vi "Main FPGA.vi"() -> ()   [LabVIEW 2015]
uses:
  Controls/FPGA_ACQTime State.ctl
  Controls/Phase State.ctl
  Controls/FPGA_Line Syn. State.ctl
  Controls/FPGA_Y AO State.ctl
  Controls/FPGA_Stimulate State.ctl
  <vilib>/Platform/TimedLoop/XDataNode/timing_clust.ctl
  <vilib>/Platform/TimedLoop/XDataNode/nitl_modes.ctl
  <vilib>/Platform/TimedLoop/XDataNode/wakeup.ctl
  Controls/FPGA_Enable Frame State.ctl
  <vilib>/rvi/Emulation/niFpgaGetClockAttributes.vi
  <vilib>/rvi/Emulation/niFpgaSctlEmulationGetInTimedLoop.vi
  <vilib>/rvi/Emulation/niFpgaEmulationReportErrorSimple.vi
  <vilib>/rvi/Emulation/niFpgaProcessEmulError.vi
  <vilib>/rvi/eio/common/nirviEmuTemplateMethod_errors.vi
  <vilib>/rvi/Emulation/niFpgaCriticalErrorInLSC.vi
  <vilib>/rvi/Memory/Memory_Emulation/nirvimemoryFastEmulation.vi
  <vilib>/rvi/Memory/Memory_Emulation/nirvimemoryEmulation.vi
  <vilib>/rvi/Emulation/niFpgaEmulationIsFPGAContextNoSignature.vi
  <vilib>/rvi/DataTransferAndStorage/Container/Common/niFpgaContainerGetUniqueNameForEmu.vi
  <vilib>/rvi/errors/nirviReportUnexpectedCaseInternalError (U32).vi
  <vilib>/rvi/interface/RandomDataEmulation/niFpgaRandomDataHandleErrors.vi
  <vilib>/eio/EIONode/EIONode.xnode
  <vilib>/rvi/DataTransferAndStorage/Container/XNode/niFpgaContainer.xnode
  <vilib>/Platform/TimedLoop/XDataNode/XDataNode.xnode
  <vilib>/rvi/interface/RandomDataEmulation/nirviRandomDataFpgaReadWriteTemplate.vi
  <instrlib>/_niInstr/Basic Elements/v1/FPGA/niInstr Basic Elements v1 FPGA.lvlib
  <vilib>/Platform/TimedLoop/XDataNode/XDNodeRunTimeDep.lvlib
panel:
  in  "PMT1 Enable":bool
  in  "Vision Stimulate Value":i16
  in  "Stimulate Enable":bool
  in  "Stimulate Time":u32
  in  "Stimulate Interval":u32
  in  "Frames Befor Stimulate":u32
  out "Frame Number":u32
  out "VSYNC":bool
  out "Actual Stimulate Ticks":u32
  out "Actual Laser Intensity":i16
  in  "Actual Laser Intensity Count":u32
  out "Acutal Actual Laser Intensity Count":u32
  in  "Y Offset":i16
  in  "Point":bool
  in  "Microscope":enum16{"Miniature", "Benchtop"}(ring)
  in  "Laser Intensity Count(Ticks)":u32 caption="PMT Sensitivity Count(Ticks)"
  out "Actual Laser Intensity Count(Ticks)":u32
  out "Acq. Syn. Out":bool
  in  "X Offset":i16
  in  "Laser Intensity":i16
  in  "Threh.Low":i16
  in  "Threh.High":i16
  in  "High Dealy":u32
  in  "Low Dealy":u32
  out "Actual PMT Sensitivity Count(Ticks)":u32
  in  "PMT Sensitivity Count(Ticks)":u32
  in  "PMT Sensitivity":i16
  in  "Start Control":bool
  out "2":i16
  out "1":i16
  out "Triangle 剩余元素":u32
  out "Ramp 剩余元素":u32
  out "IDLE":bool
  out "Ramp 待读取元素数量":u32
  out "Triangle 待读取元素数量":u32
  in  "Shutter":bool
  out "Falling Detected":bool
  out "Rising Detected":bool
  in  "Phase Shift":u32
  out "Acq. Time Number":u32
  out "Line Dis.":u32
  in  "Line":u32
  in  "Ramp Step":i16
  in  "Ramp Start":i16
  in  "Triangle Min":i16
  in  "Triangle Max":i16
  out "Ramp Number":u32
  out "Ramp OutEnable":bool
  out "Laser data out":i16
  in  "FPGA Stop":bool=TRUE
  out "Actual Wave Ticks":u32
  out "Triangle OutEnable":bool
  in  "Wave Ticks":u32
  out "Triangle Number":u32
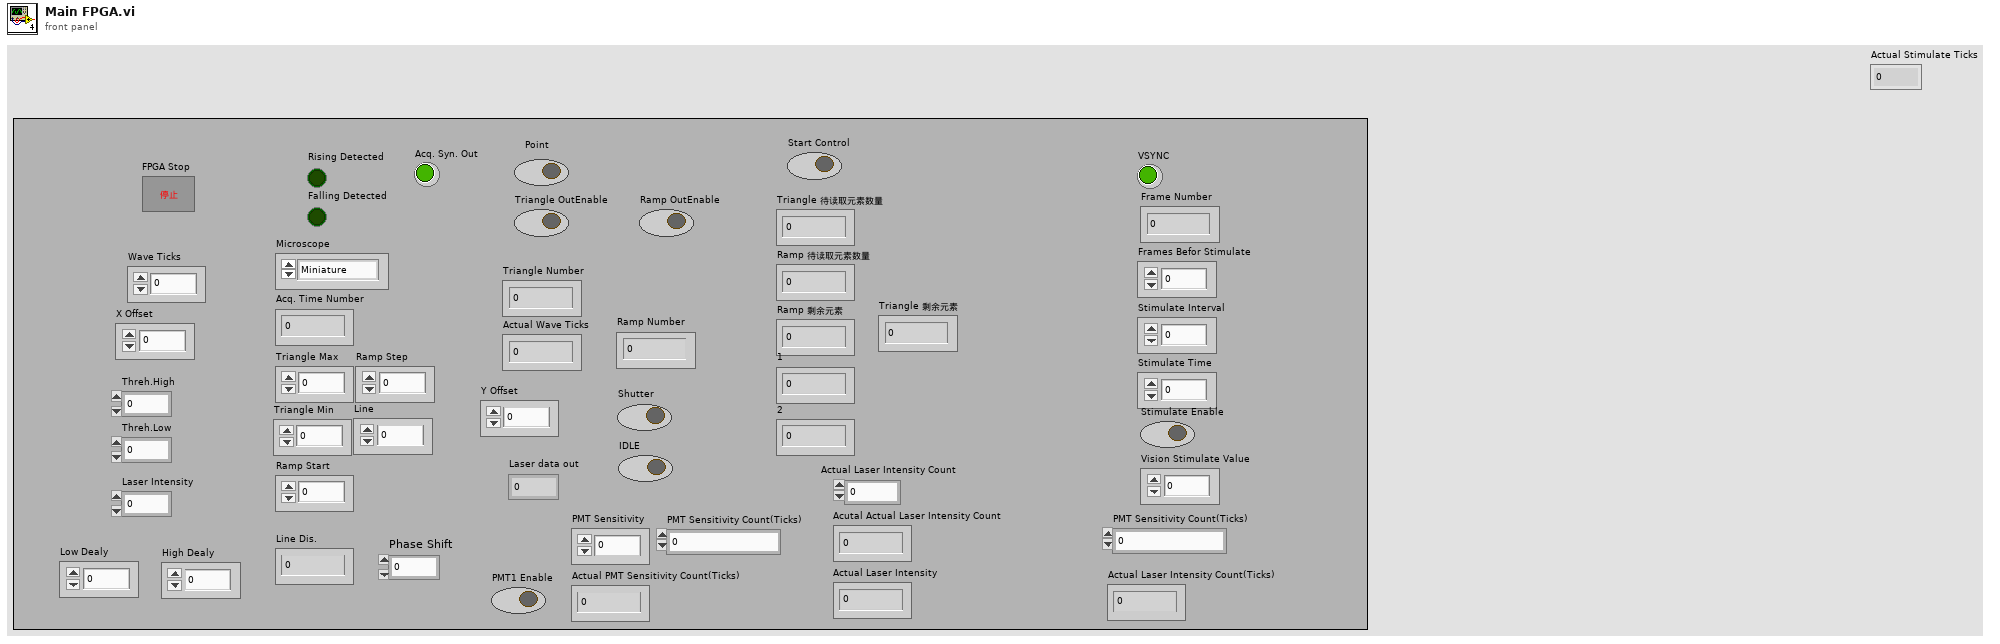
[diagram p1: front panel]
types:
  T1 = typedef "FPGA_Stimulate State.ctl" = enum16{"Wait Frame", "Frame Count", "Stiumalting", "Stiumlate Delay"}
  T2 = typedef "FPGA_Y AO State.ctl" = enum16{"Frame Start", "Framing", "Ramp"}
  T3 = typedef "FPGA_Line Syn. State.ctl" = enum16{"Wait Low", "Low Delay", "Wait High", "High Delay"}
  T4 = typedef "Phase State.ctl" = enum16{"Wait for Rising", "Wait for Falling ", "Rising Delay", "Falling Delay"}
  T5 = typedef "FPGA_ACQTime State.ctl" = enum16{"Init", "Rising Eadge", "Falling Eadge"}
  T6 = typedef "FPGA_Enable Frame State.ctl" = enum16{"Wait Enable", "Enable", "Output"}
  T7 = typedef "XDNodeRunTimeDep.lvlib/timing_clust.ctl" = cluster{"Expected End [f-1]":u64, "Actual End [f-1]":u64, "Finished Late? [f-1]":bool, "Expected End [i-1]":u64, "Actual End [i-1]":u64, "Finished Late? [i-1]":bool, "Expected Start [i]":u64, "Actual Start [i]":u64, "Expected Start [f]":u64, "Actual Start [f]":u64, "Source Name":string, "Structure Name":string, "Period":i64, "Deadline":i64, "Offset":i64, "Start":i64, "Priority":i32, "Timeout":i32, "Mode":T8, "Wakeup Reason":T9, "Error":errorcluster, "Source Type":string, "Secondary Source Type":string, "Global End Time":u64, "Global Start Time":u64, "Frame Duration":u64, "Iteration Duration":u64, "Assigned CPU":i32, "I/O Scan Engine Mode":u32}
  T8 = typedef "XDNodeRunTimeDep.lvlib/nitl_modes.ctl" = enum32{"No Change", "Process missed periods, maintain original phase", "Discard missed periods, maintain original phase", "Process missed periods, ignore original phase", "Discard missed periods, ignore original phase"}
  T9 = typedef "XDNodeRunTimeDep.lvlib/wakeup.ctl" = enum32{"Normal", "Aborted", "Asynchronous wakeup", "Timing source error", "Timed loop error", "Timeout"}
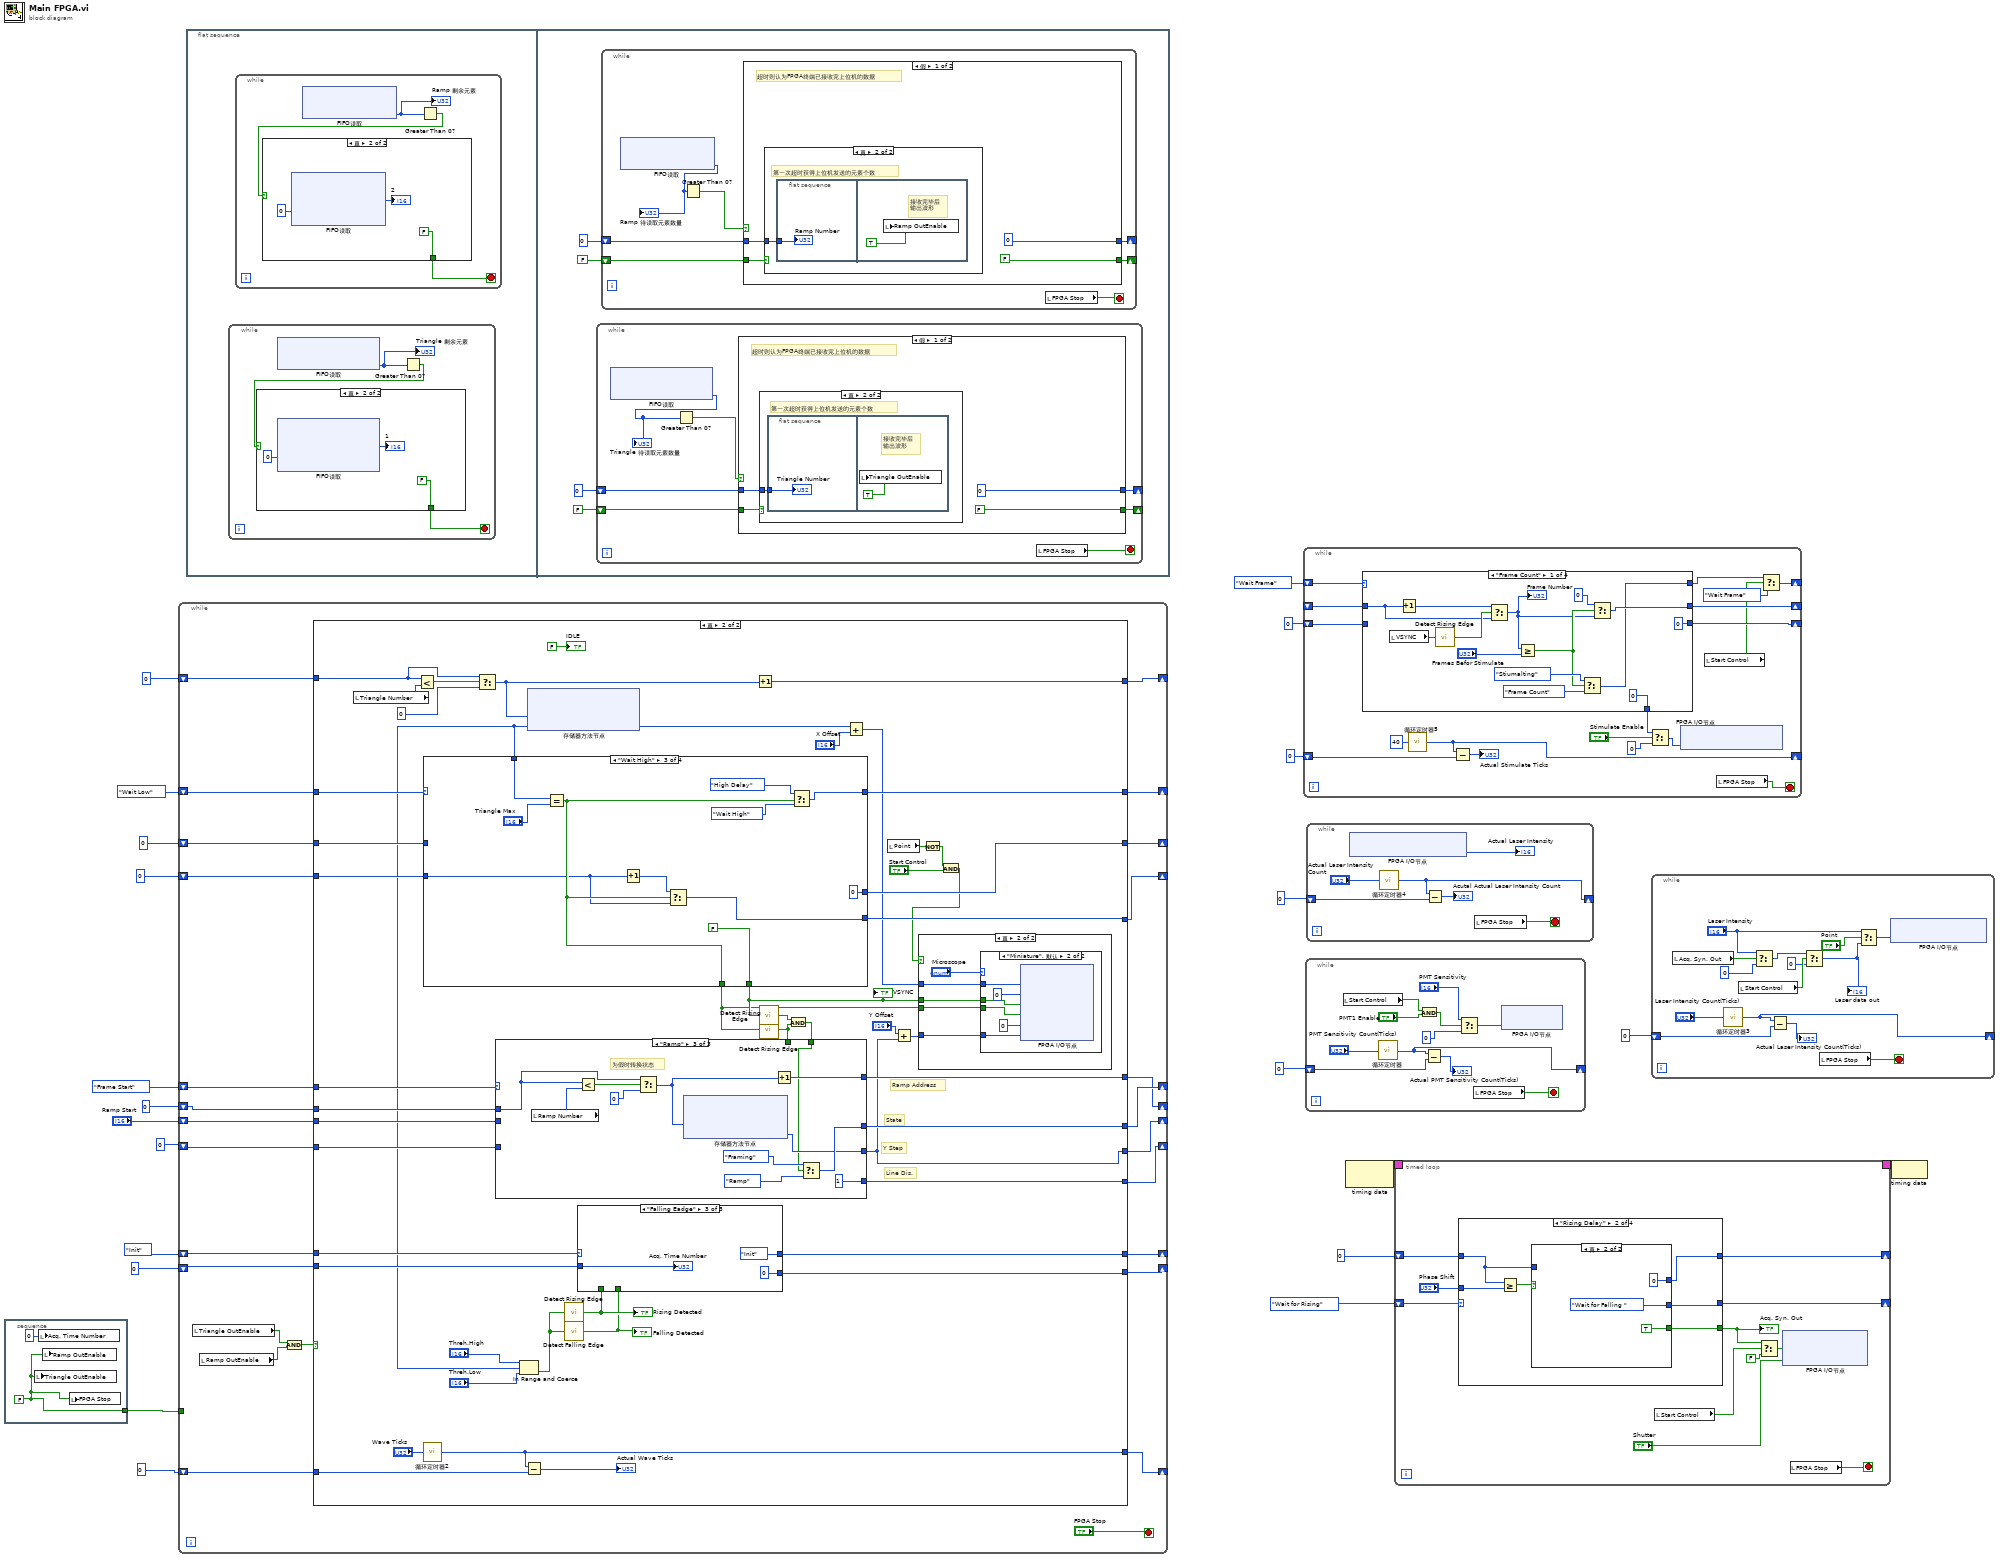
[diagram p0: block diagram]
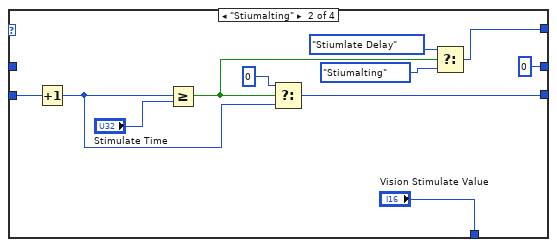
[diagram p2: hidden frame]
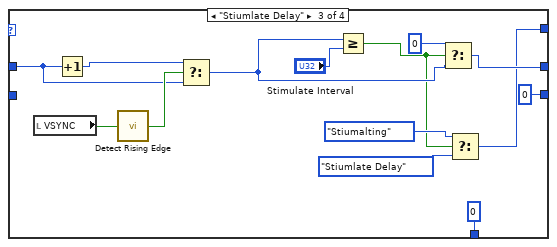
[diagram p3: hidden frame]
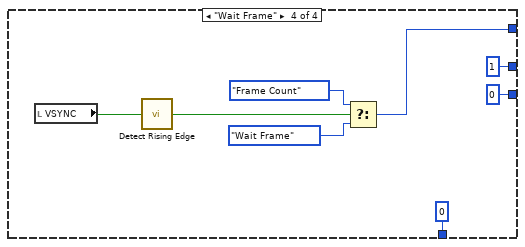
[diagram p4: hidden frame]
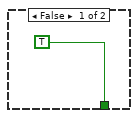
[diagram p5: hidden frame]
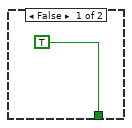
[diagram p6: hidden frame]
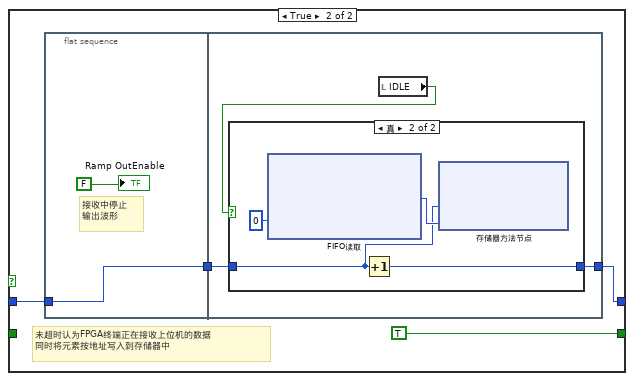
[diagram p8: hidden frame]
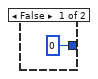
[diagram p9: hidden frame]
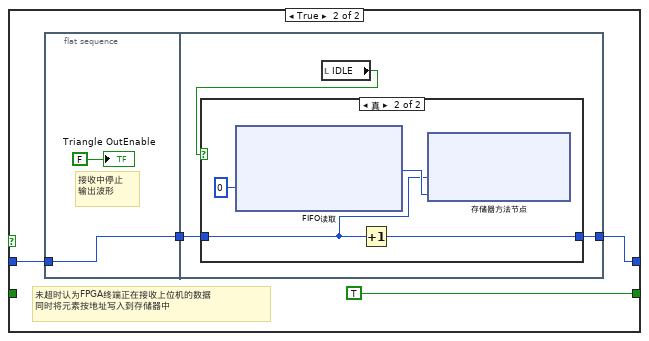
[diagram p11: hidden frame]
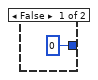
[diagram p12: hidden frame]
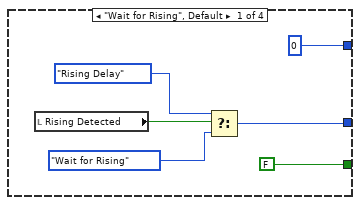
[diagram p13: hidden frame]
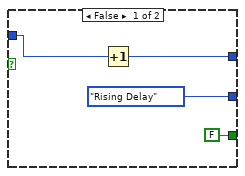
[diagram p14: hidden frame]
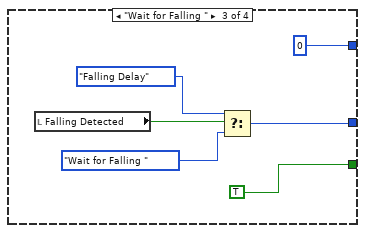
[diagram p15: hidden frame]
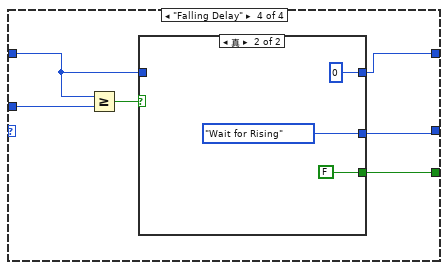
[diagram p16: hidden frame]
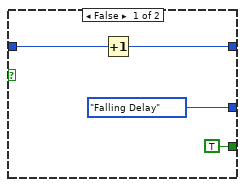
[diagram p17: hidden frame]
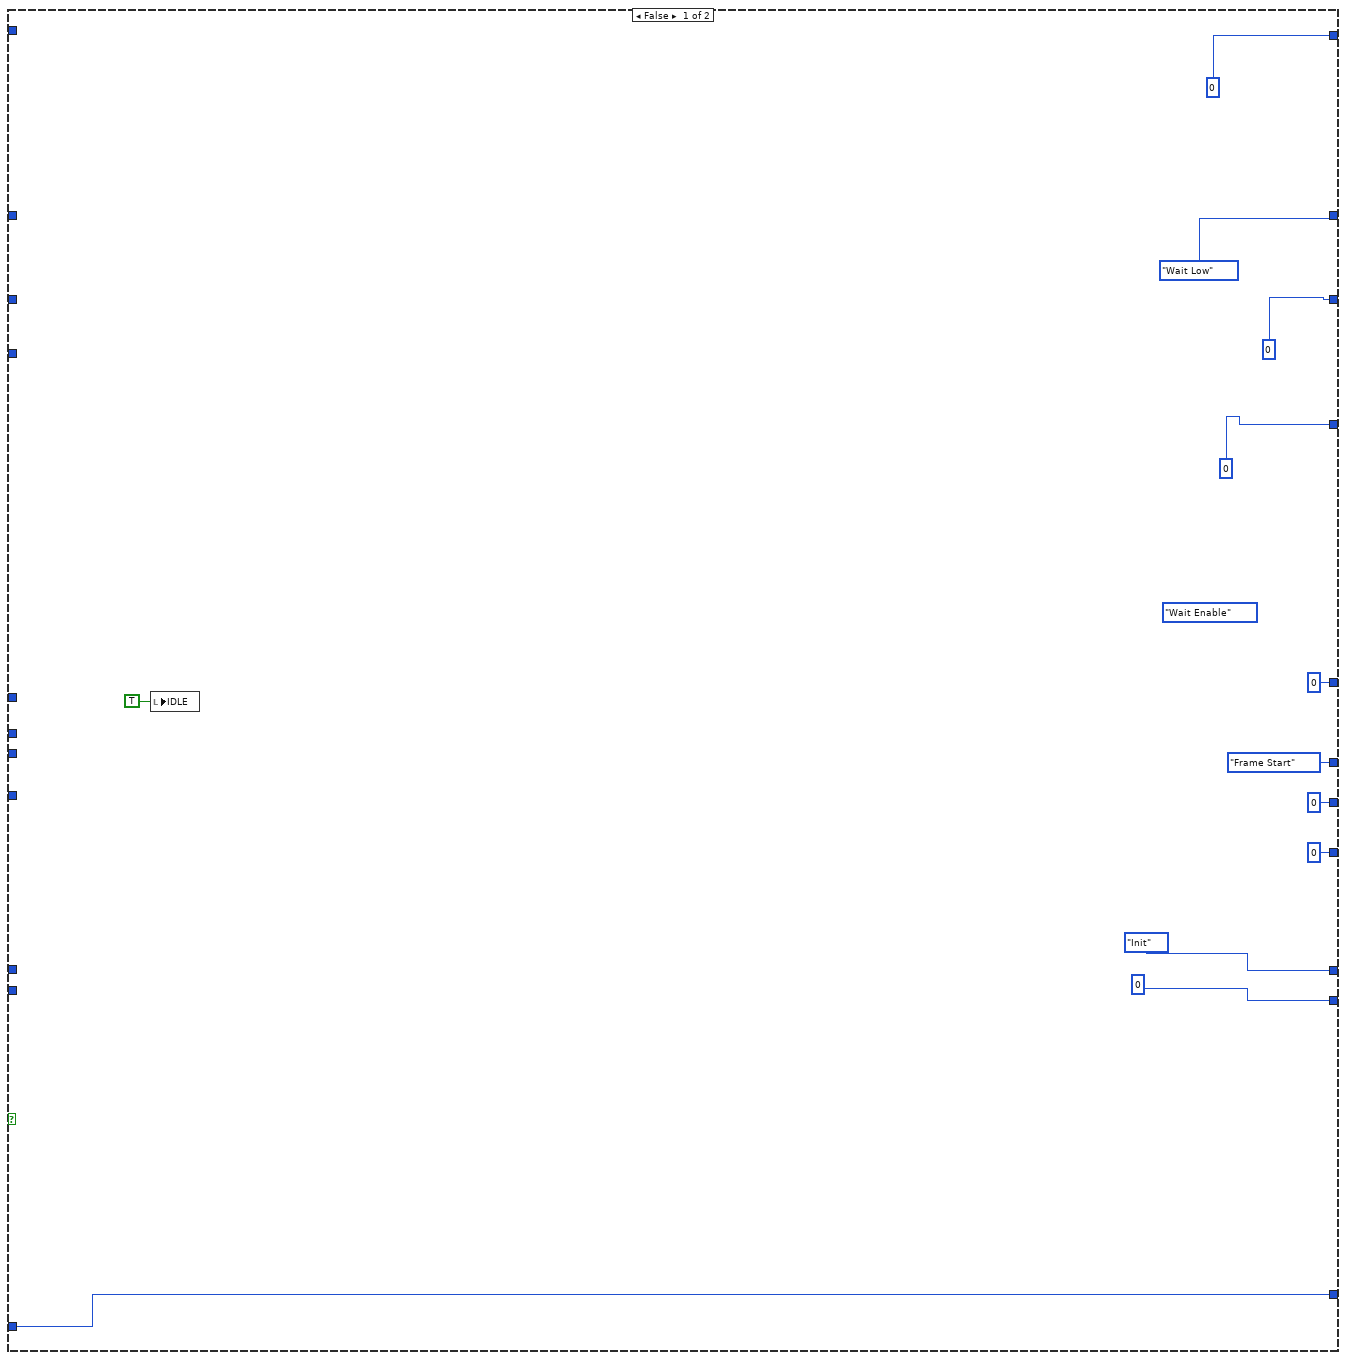
[diagram p18: hidden frame]
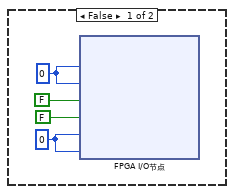
[diagram p19: hidden frame]
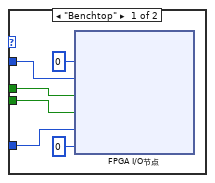
[diagram p20: hidden frame]
diagram:
  n1 = stacked-sequence {
    tunnel: [w24] -> w20
    frame #0 {
      w24 = FALSE ("FPGA Stop")
      n2 = local write "Triangle OutEnable"(w24) -> ()
      n3 = local write "Acq. Time Number"(u32 0 ("Acq. Time Number")) -> ()
      n4 = local write "Ramp OutEnable"(w24) -> ()
      n5 = local write "FPGA Stop"(w24) -> ()
    }
  }
  n6 = while {
    shift-right: [w50] -> _
    shift-left: u32 0 ("地址") -> [w49]
    shift-right: [w48] -> _
    shift-left: u32 0 ("地址") -> [w47]
    shift-right: [w37] -> _
    shift-left: FPGA_Line_Syn._State."Wait Low" ("Line Syn. State") -> [w45]
    tunnel: w20 -> [_]
    shift-right: [w40] -> _
    shift-left: FPGA_ACQTime_State."Init" ("FPGA_ACQTime State") -> [w41]
    shift-right: [w38] -> _
    shift-left: u32 0 ("地址") -> [w39]
    shift-right: [w35] -> _
    shift-left: u32 0 ("地址") -> [w36]
    shift-right: [w33] -> _
    shift-left: u32 0 ("地址") -> [w34]
    shift-right: [w31] -> _
    shift-left: FPGA_Y_AO_State."Frame Start" ("Y/AO State") -> [w32]
    shift-right: [w28] -> _
    shift-left: "Ramp Start" -> [w30]
    shift-right: [w27] -> _
    shift-left: u32 0 ("地址") -> [w29]
    shift-right: [w25] -> _
    shift-left: u32 0 ("地址") -> [w26]
    stop <- "FPGA Stop" stop-if-true
    n7 = local read "Triangle OutEnable"() -> (w44:bool)
    n8 = local read "Ramp OutEnable"() -> (w43:bool)
    n9 = And(x=w44, y=w43) -> (x .and. y?=w42:bool)
    n10 = case shown="真" w42 {
      tunnel: [u32 0 w92] -> w50
      tunnel: w49 -> [_ w110]
      tunnel: [w61 w105] -> w48
      tunnel: w47 -> [w61 w104]
      tunnel: w45 -> [_ w102]
      tunnel: w41 -> [_ w100]
      tunnel: [FPGA_ACQTime_State."Init" ("FPGA_ACQTime State") w99] -> w40
      tunnel: w39 -> [_ w98]
      tunnel: [u32 0 ("地址") w97] -> w38
      tunnel: [FPGA_Line_Syn._State."Wait Low" ("Line Syn. State") w91] -> w37
      tunnel: w36 -> [_ w90]
      tunnel: [u32 0 ("地址") w89] -> w35
      tunnel: w34 -> [_ w88]
      tunnel: [u32 0 ("地址") w87] -> w33
      tunnel: w32 -> [_ w86]
      tunnel: [FPGA_Y_AO_State."Frame Start" ("Y/AO State") w85] -> w31
      tunnel: w30 -> [_ w84]
      tunnel: w29 -> [_ w83]
      tunnel: [i16 0 ("数据") w68] -> w28
      tunnel: [u32 0 ("地址") w82] -> w27
      tunnel: w26 -> [_ w81]
      tunnel: [u32 0 w80] -> w25
      frame False {
        (unwired) FPGA_Enable_Frame_State."Wait Enable" ("Enable Frame State")
        n11 = local write "IDLE"(TRUE ("BUSY")) -> ()
      }
      frame True {
        # "Line Dis."
        # "Y Step"
        # "Ramp Address"
        # "State"
        n12 = local read "Triangle Number"() -> (w106:u32)
        n13 = Less?(x=w110, y=w106) -> (x < y?=w108:bool)
        n14 = call "循环定时器2"("Count(Ticks)"="Wave Ticks") -> ("Tick Count(Ticks)"=w105:u32)
        n15 = Select(t=w110, s=w108, f=u32 0 ("地址")) -> (s? t:f=w101:u32)
        n16 = Subtract(x=w105, y=w104) -> (x-y=→"Actual Wave Ticks":u32)
        n17 = xnode ("存储器方法节点")("地址"=w101) -> ("数据"=w72:i16)  [unwired: 1 in, 1 out]
        n18 = case shown="\"Wait High\"" w102 {
          tunnel: w72 -> [w194 _ w219 _]
          tunnel: [w191 w205 w217 w230] -> w91
          tunnel: w90 -> [_ w208 _ w233]
          tunnel: [w180 TRUE ("Start") w210 TRUE ("Start")] -> w63
          tunnel: [u32 0 ("地址") w202 u32 0 ("地址") w226] -> w89
          tunnel: w88 -> [w182 w195 w209 w221]
          tunnel: [w185 w196 FALSE ("f") FALSE ("Start")] -> w78
          tunnel: [w184 w195 w212 w225] -> w87
          frame "Wait Low", Default {
            n19 = Increment(x=w182) -> (x+1=w183:u32)
            n20 = Equal?(x=w194, y="Triangle Min") -> (x = y?=w180:bool)
            n21 = Select(t=w183, s=w180, f=w182) -> (s? t:f=w184:u32)
            n22 = Equal?(x=w184, y=u32 1) -> (x = y?=w187:bool)
            n23 = Select(t=TRUE ("f"), s=w187, f=FALSE) -> (s? t:f=w185:bool)
            n24 = Select(t=FPGA_Line_Syn._State."Low Delay" ("Line Syn. State"), s=w180, f=FPGA_Line_Syn._State."Wait Low" ("Line Syn. State")) -> (s? t:f=w191:T3)
          }
          frame "Low Delay" {
            n25 = Increment(x=w208) -> (x+1=w202:u32)
            n26 = Equal?(x=w195, y=u32 1) -> (x = y?=w198:bool)
            n27 = Greater Or Equal?(x=w202, y="Low Dealy") -> (x >= y?=w203:bool)
            n28 = Select(t=TRUE ("f"), s=w198, f=FALSE) -> (s? t:f=w196:bool)
            n29 = Select(t=FPGA_Line_Syn._State."Wait High" ("Line Syn. State"), s=w203, f=FPGA_Line_Syn._State."Low Delay" ("Line Syn. State")) -> (s? t:f=w205:T3)
          }
          frame "Wait High" {
            n30 = Equal?(x=w219, y="Triangle Max") -> (x = y?=w210:bool)
            n31 = Increment(x=w209) -> (x+1=w211:u32)
            n32 = Select(t=w211, s=w210, f=w209) -> (s? t:f=w212:u32)
            n33 = Select(t=FPGA_Line_Syn._State."High Delay" ("Line Syn. State"), s=w210, f=FPGA_Line_Syn._State."Wait High" ("Line Syn. State")) -> (s? t:f=w217:T3)
          }
          frame "High Delay" {
            n34 = Increment(x=w233) -> (x+1=w226:u32)
            n35 = Greater Or Equal?(x=w221, y="Line") -> (x >= y?=w223:bool)
            n36 = Greater Or Equal?(x=w226, y="High Dealy") -> (x >= y?=w228:bool)
            n37 = Select(t=u32 0 ("地址"), s=w223, f=w221) -> (s? t:f=w225:u32)
            n38 = Select(t=FPGA_Line_Syn._State."Wait Low" ("Line Syn. State"), s=w228, f=FPGA_Line_Syn._State."High Delay" ("Line Syn. State")) -> (s? t:f=w230:T3)
          }
        }
        "VSYNC" <- w78
        n39 = In Range and Coerce(upper limit="Threh.High", x=w72, lower limit="Threh.Low") -> (In Range?=w95:bool)  [unwired: 1 out]
        n40 = call <instrlib>:"Detect Rising Edge.vi"("signal"=w95) -> ("edge detected"=w96:bool)  [unwired: 14 in]
        "Rising Detected" <- w96
        n41 = call <instrlib>:"Detect Falling Edge.vi"("signal"=w95) -> ("edge detected"=w94:bool)  [unwired: 14 in]
        "Falling Detected" <- w94
        n42 = case shown="\"Falling Eadge\"" w100 {
          tunnel: w96 -> [w170 _ _]
          tunnel: [w169 w171 FPGA_ACQTime_State."Init" ("FPGA_ACQTime State")] -> w99
          tunnel: w94 -> [_ w174 _]
          tunnel: w98 -> [w166 w173 w179]
          tunnel: [w166 w172 u32 0] -> w97
          frame "Init", Default {
            n43 = Select(t=FPGA_ACQTime_State."Rising Eadge" ("FPGA_ACQTime State"), s=w170, f=FPGA_ACQTime_State."Init" ("FPGA_ACQTime State")) -> (s? t:f=w169:T5)
          }
          frame "Rising Eadge" {
            n44 = Increment(x=w173) -> (x+1=w172:u32)
            n45 = Select(t=FPGA_ACQTime_State."Falling Eadge" ("FPGA_ACQTime State"), s=w174, f=FPGA_ACQTime_State."Rising Eadge" ("FPGA_ACQTime State")) -> (s? t:f=w171:T5)
          }
          frame "Falling Eadge" {
            "Acq. Time Number" <- w179
          }
        }
        n46 = Increment(x=w101) -> (x+1=w92:u32)
        n47 = call <instrlib>:"Detect Rising Edge.vi"("signal"=w78) -> ("edge detected"=w79:bool)  [unwired: 14 in]
        n48 = call <instrlib>:"Detect Rising Edge.vi"("signal"=w63) -> ("edge detected"=w76:bool)  [unwired: 14 in]
        n49 = And(x=w79, y=w76) -> (x .and. y?=w77:bool)
        n50 = case shown="\"Ramp\"" w86 {
          tunnel: [w134 w147 w158] -> w85
          tunnel: w84 -> [_ w139 _]
          tunnel: w83 -> [_ w151 _]
          tunnel: [w133 w142 w156] -> w68
          tunnel: [u32 1 ("地址") w146 u32 1 ("地址")] -> w82
          tunnel: w81 -> [_ _ w164]
          tunnel: [u32 0 u32 0 w163] -> w80
          tunnel: w77 -> [w132 _ w155]
          tunnel: w76 -> [_ w143 _]
          frame "Frame Start", Default {
            n51 = local read "Ramp Start"() -> (w133:i16)
            n52 = Select(t=FPGA_Y_AO_State."Framing" ("Y/AO State"), s=w132, f=FPGA_Y_AO_State."Frame Start" ("Y/AO State")) -> (s? t:f=w134:T2)
          }
          frame "Framing" {
            # "最后一个不\n增加step电压"
            n53 = Increment(x=w151) -> (x+1=w152:u32)
            n54 = Add(x="Ramp Step", y=w139) -> (x+y=w150:i16)
            n55 = local read "Line"() -> (w144:u32)
            n56 = Select(t=w150, s=w143, f=w139) -> (s? t:f=w141:i16)
            n57 = Select(t=w152, s=w143, f=w151) -> (s? t:f=w146:u32)
            "Line Dis." <- w146
            n58 = Greater Or Equal?(x=w146, y=w144) -> (x >= y?=w140:bool)
            n59 = Select(t=FPGA_Y_AO_State."Ramp" ("Y/AO State"), s=w140, f=FPGA_Y_AO_State."Framing" ("Y/AO State")) -> (s? t:f=w147:T2)
            n60 = Select(t=w139, s=w140, f=w141) -> (s? t:f=w142:i16)
          }
          frame "Ramp" {
            # "为假时转换状态"
            n61 = local read "Ramp Number"() -> (w154:u32)
            n62 = Less?(x=w164, y=w154) -> (x < y?=w160:bool)
            n63 = Select(t=w164, s=w160, f=u32 0 ("地址")) -> (s? t:f=w162:u32)
            n64 = xnode ("存储器方法节点")("地址"=w162) -> ("数据"=w156:i16)  [unwired: 1 in, 1 out]
            n65 = Increment(x=w162) -> (x+1=w163:u32)
            n66 = Select(t=FPGA_Y_AO_State."Framing" ("Y/AO State"), s=w155, f=FPGA_Y_AO_State."Ramp" ("Y/AO State")) -> (s? t:f=w158:T2)
          }
        }
        n67 = Add(x=w72, y="X Offset") -> (x+y=w73:i16)
        n68 = local read "Point"() -> (w66:bool)
        n69 = Add(x="Y Offset", y=w68) -> (x+y=w70:i16)
        n70 = Not(x=w66) -> (.not. x?=w65:bool)
        n71 = And(x=w65, y="Start Control") -> (x .and. y?=w64:bool)
        n72 = case shown="真" w64 {
          tunnel: w78 -> [_ w119]
          tunnel: w63 -> [_ w118]
          tunnel: w70 -> [_ w117]
          tunnel: w73 -> [_ w116]
          frame False {
            w114 = i16 0 ("X/AO0")
            w111 = i16 0 ("Y/AO1")
            n73 = xnode "FPGA I/O节点"("X-M/AO0"=w114, "X-S/AO6"=w114, "VSYNC/DIO2"=FALSE, "HSYNC/DIO1"=FALSE, "Y-S/AO7"=w111, "Y-M/AO1"=w111) -> ()  [unwired: 6 in, 6 out]
          }
          frame True {
            n74 = case shown="\"Miniature\", 默认" "Microscope" {
              tunnel: w119 -> [w125 w131]
              tunnel: w118 -> [w124 w130]
              tunnel: w117 -> [w123 w128]
              tunnel: w116 -> [w122 w126]
              frame "Benchtop" {
                n75 = xnode "FPGA I/O节点"("X-M/AO0"=i16 0, "X-S/AO6"=w122, "VSYNC/DIO2"=w125, "HSYNC/DIO1"=w124, "Y-S/AO7"=w123, "Y-M/AO1"=i16 0) -> ()  [unwired: 6 in, 6 out]
              }
              frame "Miniature", Default {
                n76 = xnode "FPGA I/O节点"("X-M/AO0"=w126, "X-S/AO6"=i16 0 ("X-M/AO0"), "VSYNC/DIO2"=w131, "HSYNC/DIO1"=w130, "Y-S/AO7"=i16 0 ("Y-M/AO1"), "Y-M/AO1"=w128) -> ()  [unwired: 6 in, 6 out]
              }
            }
          }
        }
        "IDLE" <- FALSE ("执行")
      }
    }
  }
  n77 = flat-sequence {
    frame #0 {
      n78 = while {
        stop <- w241 stop-if-true
        n79 = xnode ("FIFO读取")() -> ("待读取元素数量"=w243:u32)  [unwired: 1 in, 1 out]
        "Triangle 剩余元素" <- w243
        n80 = Greater Than 0?(x=w243) -> (x > 0?=w242:bool)
        n81 = case shown="真" w242 {
          tunnel: [TRUE ("执行") FALSE ("输出波形")] -> w241
          frame False {
          }
          frame True {
            n82 = xnode ("FIFO读取")("超时"=0) -> ("元素"=→"1":i16)  [unwired: 1 in, 2 out]
          }
        }
      }
      n83 = while {
        stop <- w234 stop-if-true
        n84 = xnode ("FIFO读取")() -> ("待读取元素数量"=w236:u32)  [unwired: 1 in, 1 out]
        "Ramp 剩余元素" <- w236
        n85 = Greater Than 0?(x=w236) -> (x > 0?=w235:bool)
        n86 = case shown="真" w235 {
          tunnel: [TRUE ("执行") FALSE ("执行")] -> w234
          frame False {
          }
          frame True {
            n87 = xnode ("FIFO读取")("超时"=0) -> ("元素"=→"2":i16)  [unwired: 1 in, 2 out]
          }
        }
      }
    }
    frame #1 {
      n88 = while {
        shift-right: [w285] -> _
        shift-left: u32 0 ("地址") -> [w286]
        shift-right: [w283] -> _
        shift-left: FALSE ("执行") -> [w284]
        stop <- w282 stop-if-true
        n89 = xnode ("FIFO读取")() -> ("待读取元素数量"=w281:u32)  [unwired: 1 in, 1 out]
        "Triangle 待读取元素数量" <- w281
        n90 = Greater Than 0?(x=w281) -> (x > 0?=w280:bool)
        n91 = case shown="假" w280 {
          tunnel: w286 -> [w288 w295]
          tunnel: [u32 0 w294] -> w285
          tunnel: w284 -> [w289 _]
          tunnel: [FALSE TRUE] -> w283
          frame False {
            # "超时则认为FPGA终端已接收完上位机的数据"
            n92 = case shown="真" w289 {
              tunnel: w288 -> [_ w291]
              frame False {
              }
              frame True {
                # "第一次超时获得上位机发送的元素个数"
                n93 = flat-sequence {
                  tunnel: w291 -> [w292]
                  frame #0 {
                    "Triangle Number" <- w292
                  }
                  frame #1 {
                    # "接收完毕后\n输出波形"
                    n94 = local write "Triangle OutEnable"(TRUE ("执行")) -> ()
                  }
                }
              }
            }
          }
          frame True {
            # "未超时认为FPGA终端正在接收上位机的数据\n同时将元素按地址写入到存储器中"
            n95 = flat-sequence {
              tunnel: [w298] -> w296
              tunnel: w295 -> [w298]
              tunnel: w296 -> [w301]
              tunnel: [w300] -> w294
              frame #0 {
                # "接收中停止\n输出波形"
                "Triangle OutEnable" <- FALSE ("输出波形")
              }
              frame #1 {
                n96 = local read "IDLE"() -> (w302:bool)
                n97 = case shown="真" w302 {
                  tunnel: w301 -> [_ w304]
                  tunnel: [u32 0 w305] -> w300
                  frame False {
                  }
                  frame True {
                    n98 = xnode ("FIFO读取")("超时"=0) -> ("元素"=w306:i16)  [unwired: 1 in, 2 out]
                    n99 = Increment(x=w304) -> (x+1=w305:u32)
                    n100 = xnode ("存储器方法节点")("地址"=w304, "数据"=w306) -> ()  [unwired: 1 in, 1 out]
                  }
                }
              }
            }
          }
        }
        n101 = local read "FPGA Stop"() -> (w282:bool)
      }
      n102 = while {
        shift-right: [w257] -> _
        shift-left: u32 0 ("地址") -> [w258]
        shift-right: [w255] -> _
        shift-left: FALSE ("执行") -> [w256]
        stop <- w254 stop-if-true
        n103 = xnode ("FIFO读取")() -> ("待读取元素数量"=w252:u32)  [unwired: 1 in, 1 out]
        "Ramp 待读取元素数量" <- w252
        n104 = Greater Than 0?(x=w252) -> (x > 0?=w253:bool)
        n105 = case shown="假" w253 {
          tunnel: w258 -> [w260 w267]
          tunnel: [u32 0 w266] -> w257
          tunnel: w256 -> [w261 _]
          tunnel: [FALSE TRUE] -> w255
          frame False {
            # "超时则认为FPGA终端已接收完上位机的数据"
            n106 = case shown="真" w261 {
              tunnel: w260 -> [_ w263]
              frame False {
              }
              frame True {
                # "第一次超时获得上位机发送的元素个数"
                n107 = flat-sequence {
                  tunnel: w263 -> [w264]
                  frame #0 {
                    "Ramp Number" <- w264
                  }
                  frame #1 {
                    # "接收完毕后\n输出波形"
                    n108 = local write "Ramp OutEnable"(TRUE ("执行")) -> ()
                  }
                }
              }
            }
          }
          frame True {
            # "未超时认为FPGA终端正在接收上位机的数据\n同时将元素按地址写入到存储器中"
            n109 = flat-sequence {
              tunnel: [w270] -> w268
              tunnel: w267 -> [w270]
              tunnel: w268 -> [w273]
              tunnel: [w272] -> w266
              frame #0 {
                # "接收中停止\n输出波形"
                "Ramp OutEnable" <- FALSE ("输出波形")
              }
              frame #1 {
                n110 = local read "IDLE"() -> (w274:bool)
                n111 = case shown="真" w274 {
                  tunnel: w273 -> [_ w276]
                  tunnel: [u32 0 w277] -> w272
                  frame False {
                  }
                  frame True {
                    n112 = xnode ("FIFO读取")("超时"=0) -> ("元素"=w278:i16)  [unwired: 1 in, 2 out]
                    n113 = Increment(x=w276) -> (x+1=w277:u32)
                    n114 = xnode ("存储器方法节点")("地址"=w276, "数据"=w278) -> ()  [unwired: 1 in, 1 out]
                  }
                }
              }
            }
          }
        }
        n115 = local read "FPGA Stop"() -> (w254:bool)
      }
    }
  }
  n116 = while {
    shift-right: [w324] -> _
    shift-left: u32 0 ("地址") -> [w325]
    shift-right: [w315] -> _
    shift-left: FPGA_Stimulate_State."Wait Frame" ("Stimulate State") -> [w322]
    shift-right: [w320] -> _
    shift-left: _ -> [w321]
    shift-right: [w316] -> _
    shift-left: u32 0 ("地址") -> [w319]
    stop <- w317 stop-if-true
    n117 = case shown="\"Frame Count\"" w322 {
      tunnel: [w328 w345 w354 w370] -> w314
      tunnel: w321 -> [w336 _ w359 _]
      tunnel: [w330 u32 0 ("地址") w362 u32 1 ("地址")] -> w320
      tunnel: [i16 0 ("地址") "Vision Stimulate Value" i16 0 ("地址") i16 0 ("地址")] -> w309
      tunnel: w319 -> [_ w350 _ _]
      tunnel: [u32 0 ("地址") w342 u32 0 ("地址") u32 0 ("地址")] -> w316
      frame "Frame Count" {
        n118 = local read "VSYNC"() -> (w339:bool)
        n119 = Increment(x=w336) -> (x+1=w337:u32)
        n120 = call <instrlib>:"Detect Rising Edge.vi"("signal"=w339) -> ("edge detected"=w338:bool)  [unwired: 14 in]
        n121 = Select(t=w337, s=w338, f=w336) -> (s? t:f=w331:u32)
        "Frame Number" <- w331
        n122 = Greater Or Equal?(x=w331, y="Frames Befor Stimulate") -> (x >= y?=w332:bool)
        n123 = Select(t=FPGA_Stimulate_State."Stiumalting" ("Stimulate State"), s=w332, f=FPGA_Stimulate_State."Frame Count" ("Stimulate State")) -> (s? t:f=w328:T1)
        n124 = Select(t=u32 0, s=w332, f=w331) -> (s? t:f=w330:u32)
      }
      frame "Stiumalting" {
        n125 = Increment(x=w350) -> (x+1=w347:u32)
        n126 = Greater Or Equal?(x=w347, y="Stimulate Time") -> (x >= y?=w346:bool)
        n127 = Select(t=u32 0 ("地址"), s=w346, f=w347) -> (s? t:f=w342:u32)
        n128 = Select(t=FPGA_Stimulate_State."Stiumlate Delay" ("Stimulate State"), s=w346, f=FPGA_Stimulate_State."Stiumalting" ("Stimulate State")) -> (s? t:f=w345:T1)
      }
      frame "Stiumlate Delay" {
        n129 = local read "VSYNC"() -> (w361:bool)
        n130 = Increment(x=w359) -> (x+1=w358:u32)
        n131 = call <instrlib>:"Detect Rising Edge.vi"("signal"=w361) -> ("edge detected"=w360:bool)  [unwired: 14 in]
        n132 = Select(t=w358, s=w360, f=w359) -> (s? t:f=w357:u32)
        n133 = Greater Or Equal?(x=w357, y="Stimulate Interval") -> (x >= y?=w353:bool)
        n134 = Select(t=u32 0 ("地址"), s=w353, f=w357) -> (s? t:f=w362:u32)
        n135 = Select(t=FPGA_Stimulate_State."Stiumalting" ("Stimulate State"), s=w353, f=FPGA_Stimulate_State."Stiumlate Delay" ("Stimulate State")) -> (s? t:f=w354:T1)
      }
      frame "Wait Frame" {
        n136 = local read "VSYNC"() -> (w372:bool)
        n137 = call <instrlib>:"Detect Rising Edge.vi"("signal"=w372) -> ("edge detected"=w371:bool)  [unwired: 14 in]
        n138 = Select(t=FPGA_Stimulate_State."Frame Count" ("Stimulate State"), s=w371, f=FPGA_Stimulate_State."Wait Frame" ("Stimulate State")) -> (s? t:f=w370:T1)
      }
    }
    n139 = call "循环定时器5"("Count(Ticks)"=u32 40) -> ("Tick Count(Ticks)"=w324:u32)
    n140 = Subtract(x=w324, y=w325) -> (x-y=→"Actual Stimulate Ticks":u32)
    n141 = Select(t=w309, s="Stimulate Enable", f=i16 0 ("地址")) -> (s? t:f=w310:i16)
    n142 = xnode "FPGA I/O节点"("Vision Stimulate/AO5"=w310) -> ()  [unwired: 1 in, 1 out]
    n143 = local read "Start Control"() -> (w313:bool)
    n144 = local read "FPGA Stop"() -> (w317:bool)
    n145 = Select(t=w314, s=w313, f=FPGA_Stimulate_State."Wait Frame" ("Stimulate State")) -> (s? t:f=w315:T1)
  }
  n146 = while {
    shift-right: [w380] -> _
    shift-left: u32 0 ("地址") -> [w381]
    stop <- w383 stop-if-true
    n147 = local read "Start Control"() -> (w375:bool)
    n148 = call "循环定时器"("Count(Ticks)"="PMT Sensitivity Count(Ticks)") -> ("Tick Count(Ticks)"=w380:u32)
    n149 = And(x=w375, y="PMT1 Enable") -> (x .and. y?=w373:bool)
    n150 = Subtract(x=w380, y=w381) -> (x-y=→"Actual PMT Sensitivity Count(Ticks)":u32)
    n151 = Select(t="PMT Sensitivity", s=w373, f=i16 0) -> (s? t:f=w378:i16)
    n152 = local read "FPGA Stop"() -> (w383:bool)
    n153 = xnode "FPGA I/O节点"("PMT/AO3"=w378) -> ()  [unwired: 1 in, 1 out]
  }
  n154 = while {
    shift-right: [w386] -> _
    shift-left: u32 0 ("地址") -> [w387]
    stop <- w389 stop-if-true
    n155 = xnode "FPGA I/O节点"() -> ("Actual Laser Intensity/AI0"=→"Actual Laser Intensity":i16)  [unwired: 1 in, 1 out]
    n156 = call "循环定时器4"("Count(Ticks)"="Actual Laser Intensity Count") -> ("Tick Count(Ticks)"=w386:u32)
    n157 = Subtract(x=w386, y=w387) -> (x-y=→"Acutal Actual Laser Intensity Count":u32)
    n158 = local read "FPGA Stop"() -> (w389:bool)
  }
  n159 = node-c288() -> (w17:T7)  [unwired: 1 in]
  n160 = timed-loop {
    timing: w17 -> [_]
    timing-out: [_] -> w16
    shift-right: [w397] -> _
    shift-left: u32 0 ("地址") -> [w399]
    shift-right: [w396] -> _
    shift-left: Phase_State."Wait for Rising" ("Phase State") -> [w398]
    stop <- w395 stop-if-true
    n161 = case shown="\"Rising Delay\"" w398 {
      tunnel: [w405 w408 w423 w427] -> w396
      tunnel: w399 -> [_ w411 _ w429]
      tunnel: [u32 0 w410 u32 0 w428] -> w397
      tunnel: [FALSE w409 TRUE w426] -> w392
      tunnel: "Phase Shift" -> [_ w407 _ w430]
      frame "Wait for Rising", Default {
        n162 = local read "Rising Detected"() -> (w401:bool)
        n163 = Select(t=Phase_State."Rising Delay" ("Phase State"), s=w401, f=Phase_State."Wait for Rising" ("Phase State")) -> (s? t:f=w405:T4)
      }
      frame "Rising Delay" {
        n164 = Greater Or Equal?(x=w411, y=w407) -> (x >= y?=w412:bool)
        n165 = case shown="真" w412 {
          tunnel: w411 -> [w416 _]
          tunnel: [w415 u32 0] -> w410
          tunnel: [FALSE TRUE] -> w409
          tunnel: [Phase_State."Rising Delay" ("Phase State") Phase_State."Wait for Falling " ("Phase State")] -> w408
          frame False {
            n166 = Increment(x=w416) -> (x+1=w415:u32)
          }
          frame True {
          }
        }
      }
      frame "Wait for Falling " {
        n167 = local read "Falling Detected"() -> (w420:bool)
        n168 = Select(t=Phase_State."Falling Delay" ("Phase State"), s=w420, f=Phase_State."Wait for Falling " ("Phase State")) -> (s? t:f=w423:T4)
      }
      frame "Falling Delay" {
        n169 = Greater Or Equal?(x=w429, y=w430) -> (x >= y?=w431:bool)
        n170 = case shown="真" w431 {
          tunnel: w429 -> [w435 _]
          tunnel: [w434 u32 0] -> w428
          tunnel: [TRUE FALSE] -> w426
          tunnel: [Phase_State."Falling Delay" ("Phase State") Phase_State."Wait for Rising" ("Phase State")] -> w427
          frame False {
            n171 = Increment(x=w435) -> (x+1=w434:u32)
          }
          frame True {
          }
        }
      }
    }
    "Acq. Syn. Out" <- w392
    n172 = local read "Start Control"() -> (w391:bool)
    n173 = Select(t=w392, s=w391, f=FALSE) -> (s? t:f=w393:bool)
    n174 = xnode "FPGA I/O节点"("Acqusition/DIO0"=w393, "Shutter/DIO3"="Shutter") -> ()  [unwired: 2 in, 2 out]
    n175 = local read "FPGA Stop"() -> (w395:bool)
  }
  n176 = while {
    shift-right: [w451] -> _
    shift-left: u32 0 ("地址") -> [w452]
    stop <- w454 stop-if-true
    n177 = local read "Acq. Syn. Out"() -> (w448:bool)
    n178 = call "循环定时器3"("Count(Ticks)"="Laser Intensity Count(Ticks)") -> ("Tick Count(Ticks)"=w451:u32)
    n179 = local read "Start Control"() -> (w446:bool)
    n180 = Select(t="Laser Intensity", s=w448, f=i16 0 ("Threh.Low")) -> (s? t:f=w447:i16)
    n181 = Subtract(x=w451, y=w452) -> (x-y=→"Actual Laser Intensity Count(Ticks)":u32)
    n182 = Select(t=w447, s=w446, f=i16 0) -> (s? t:f=w442:i16)
    "Laser data out" <- w442
    n183 = local read "FPGA Stop"() -> (w454:bool)
    n184 = Select(t="Laser Intensity", s="Point", f=w442) -> (s? t:f=w444:i16)
    n185 = xnode "FPGA I/O节点"("Laser Intensity/AO2"=w444) -> ()  [unwired: 1 in, 1 out]
  }
  n186 = node-c288(w16) -> ()
